vi "Remove Service.vi"(8 "error in (no error)":errorcluster, 10 "Service Type":T1, 11 "DiscoveryService in":refnum<class "DiscoveryService.lvclass">) -> (0 "error out":errorcluster, 3 "DiscoveryService out":refnum<class "DiscoveryService.lvclass">)   [LabVIEW 2020, in "Vecto.lvlib" / "DiscoveryService.lvclass"]
uses:
  DiscoveryService.lvclass
  lv-volatus/messages/ServiceType/Enumeration.ctl
  DiscoveryService.lvclass/DiscoveryService.ctl
  lv-volatus/messages/ServiceType/ServiceType.lvlib
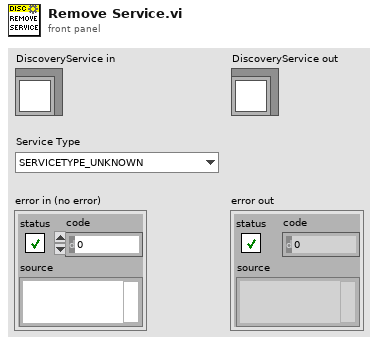
[diagram p1: front panel]
types:
  T1 = typedef "ServiceType.lvlib/Enumeration.ctl" = enum16{"SERVICETYPE_UNKNOWN", "SERVICETYPE_TCPSERVER", "SERVICETYPE_HTTPSERVER"}
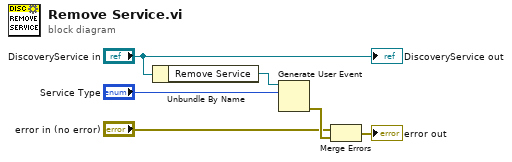
[diagram p0: block diagram]
diagram:
  n1 = Unbundle By Name("DiscoveryService in") -> ("Remove Service"=w6:refnum<user-event>)
  n2 = Generate User Event(user event=w6, event data cluster="Service Type") -> (error out=w4:errorcluster)  [unwired: 2 in, 1 out]
  n3 = Merge Errors("error in (no error)", w4) -> (→"error out":errorcluster)
  "DiscoveryService out" <- "DiscoveryService in"
